vi "EyeTrackerFPGA (host).vi"() -> ()   [LabVIEW 2014]
uses:
  <vilib>/userdefined/High Color/nirio_resource_hc.ctl
  <instrlib>/niHWS/nihws.llb/niHWS Open File Permissions ID.ctl
  <vilib>/FPGAPlugInAG/PXI-7952R/niLvFpga_Open_PXI-7952R.vi
  <vilib>/rvi/interface/common/dynamic/niFpgaDynamicAddResources.vi
  <vilib>/FPGAPlugInAG/PXI-7954R/niLvFpga_Open_PXI-7954R.vi
  <vilib>/FPGAPlugInAG/PXI-7953R/niLvFpga_Open_PXI-7953R.vi
  <vilib>/FPGAPlugInAG/Dynamic/niLvFpga_Reset_Dynamic.vi
  <vilib>/Utility/error.llb/Error Cluster From Error Code.vi
  <vilib>/rvi/errors/niLvFpgaAdjustHostInterfaceError.vi
  <vilib>/FPGAPlugInAG/Dynamic/niLvFpga_Run_Dynamic.vi
  <vilib>/LabVIEW Targets/FPGA/FlexRIO/CustomFPGAMethods/79XXR_Method_IOModuleStatusImpl.vi
  <vilib>/rvi/interface/common/niFpgaWaitOnOcc.vi
  <vilib>/DAQmx/write.llb/DAQmx Write (Analog 1D DBL NChan 1Samp).vi
  <instrlib>/niHWS/nihws.llb/niHWS Write Digital U16.vi
  <vilib>/FPGAPlugInAG/Dynamic/niLvFpga_Close_Dynamic.vi
  <vilib>/rvi/interface/nirviOpenFPGA/nirviOpenFPGA.xnode
  FPGA Bitfiles/EyeTrackerFPGA_PXI-7952R_EyeTrackerFPGA(F_6273CC10.lvbitx
  FPGA Bitfiles/EyeTrackerFPGA_PXI-7954R_EyeTrackerFPGA-7_4D2D153E.lvbitx
  FPGA Bitfiles/EyeTrackerFPGA_FPGATarget_EyeTrackerFPGA-7_1NUruOWZ7TY_7953R.lvbitx
  <vilib>/rvi/interface/nirviMethod/nirviMethod.xnode
  <vilib>/rvi/interface/nirviReadWriteControl/nirviReadWriteControl.xnode
  <vilib>/rvi/interface/nirviCloseFPGA/nirviCloseFPGA.xnode
  <vilib>/rvi/errors/niLvFpgaMergeErrorWithErrorCode.vi
  <vilib>/rvi/interface/Simulation/niFpgaSimulationCallBeginRW.vi
  NiFpgaLv.dll
  <vilib>/FPGAPlugInAG/Dynamic/niLvFpga_ReadFifo_Dynamic.vi
  <vilib>/FPGAPlugInAG/Dynamic/niLvFpga_ConfigureFifo_Dynamic.vi
  <vilib>/FPGAPlugInAG/Dynamic/niLvFpga_StartFifo_Dynamic.vi
  <resource>/objmgr/daqmx.rc
panel:
  in  "Setup":u16(ring) items=["1", "2", "3"]
  out "Analog Output Error":errorcluster
  out "Select Setup":bool=TRUE
  in  "DA Output Task":refnum<k21>="OpticalTrackerOutWithPupilSize"
  in  "Raw  Image":bool=TRUE
  out "Frame Time (x10 ns)":u32
  out "TraceDisplayLoop":i32
  out "Frame Number":u32
  out "ImageDisplayLoop":i32
  out "Text File Write Error":errorcluster
  out "AVI Write Error":errorcluster
  in  "Image Acq Rate":dbl=20.0
  in  "Calibration":bool=TRUE
  in  "RIO Device":T1="RIO0"
  in  "MinUpdatePeriod":dbl=5.0
  out "Elements Remaining":u32
  in  "Record":bool
  out "Tracking":bool
  in  "Preview Thresh":dbl
  in  "AnalogOut":bool=TRUE
  out "UpdateRate":dbl
  out "TenFrameTime":u32
  in  "MonitorDelay":u32=100
  in  "FrameRate":dbl=250.0
  in  "Track":bool
  in  "Send":bool
  in  "Command":string
  in  "Viewing Rate":dbl=5.0
  in  "EyePosition.Shift":i8
  in  "Brighten":i32=1
  in  "Threshold":u32=2800
  out "RealRate":dbl
  out "DataAvailable":u32
  out "PushedToHost":u32
  out "PushedToMem":u32
  out "BufferToHost\\Full":bool
  out "Timed Out?":bool
  out "Acq Status.FrameWidth":u32
  out "Acq Status.FrameHeight":u32
  out "ImLoop":i32
  out "MonLoop":i32
  out "Acq Control.Grab":bool
  out "Grabbing":bool
  out "Grabbed":bool
  out "Acq Control.Acq":bool
  in  "Grab":bool=TRUE
  out "Waveform Chart":cluster{dbl, dbl, dbl}[](graph)
  out "Frame Width":u32
  in  "stopped":bool
  out "DMA Write Timeout?":bool
  out "I/O Enabled?":bool
  out "Frame Num":u32
  out "Frame Height":u32
  out "Image":T2(plugin-control)
  in  "stop":bool
  out "Initialized?":bool
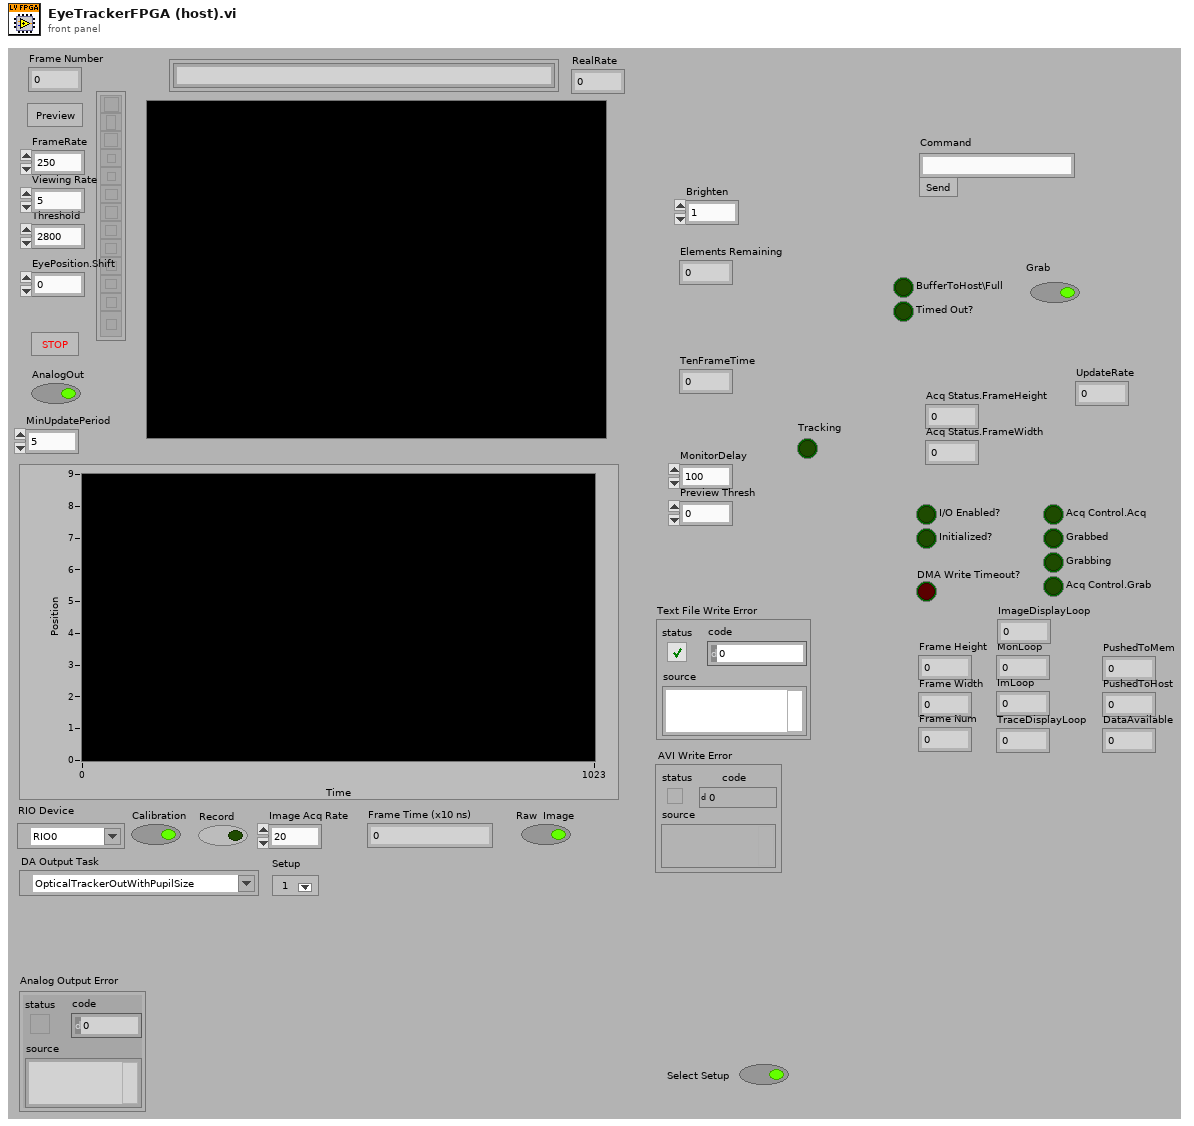
[diagram p1: front panel]
types:
  T1 = typedef "nirio_resource_hc.ctl" = tag
  T2 = typedef "IMAQ Image.ctl" = refnum<image>
  T3 = typedef "Image Type" = u32
  T4 = enum8{"Enabled", "Disabled", "Disabled and Grayed Out"}
  T5 = enum16{"open", "replace", "create", "open or create", "replace or create", "replace or create with confirmation"}
  T6 = typedef "niHWS Open File Permissions ID.ctl" = enum32{"Read Only", "Read/Write Existing", "Read/Write/Create New", "Read/Write/Create New Always"}
  T7 = typedef "AviRefnum.ctl" = refnum<k1>
  T8 = cluster{"Global Rectangle":i32[], "Contours":cluster{"Contour Type":u32, "ROI Type":u32, "Points":i32[]}[]}
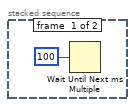
[diagram p2: hidden frame]
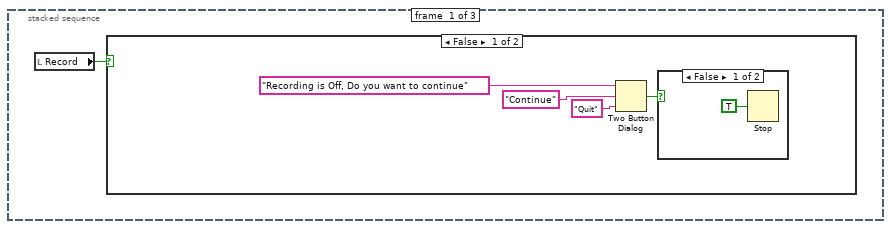
[diagram p3: hidden frame]
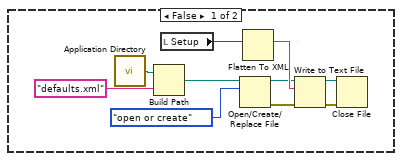
[diagram p6: hidden frame]
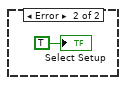
[diagram p7: hidden frame]
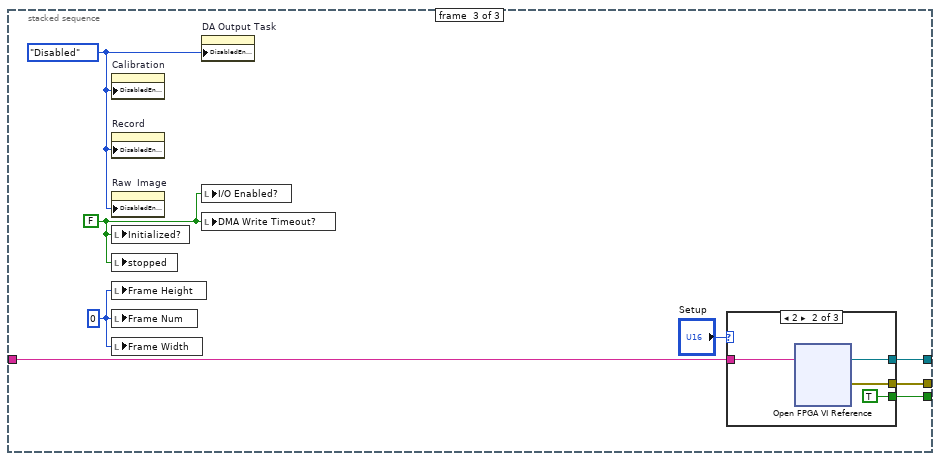
[diagram p9: hidden frame]
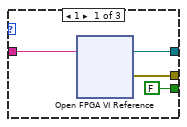
[diagram p10: hidden frame]
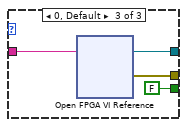
[diagram p11: hidden frame]
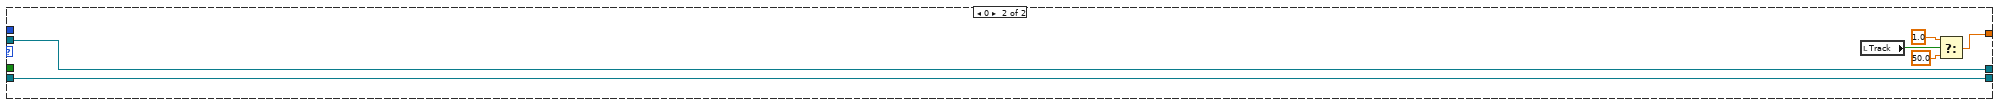
[diagram p20: hidden frame]
diagram:
  w13 = T3 0 items=["Grayscale (U8)", "Grayscale (I16)", "Grayscale (SGL)", "Complex (CSG)", "RGB (U32)", "HSL (U32)", "RGB (U64)", "Grayscale (U16)"] ("Image Type")
  w1 = T4."Enabled" ("Disabled")
  w88 = T3 0 items=["Grayscale (U8)", "Grayscale (I16)", "Grayscale (SGL)", "Complex (CSG)", "RGB (U32)", "HSL (U32)", "RGB (U64)", "Grayscale (U16)"] ("Image Type")
  # "To compile for S1:\nSelect the FPGA file from PXI-7954R\nSelect 10"
  # "relevant commands:\nsot 80 - 80 MB/s\nssf 500 - set frame rate\nset 5000 - set exposure time\nwse 0 1 x1 y1 x2 y2 - set window"
  # "Merge any errors.\nCleanup the image.\nClose the FPGA reference.\nDisplay any errors."
  # "Send software triggers as requested and monitor the acquisition status."
  # "Configure the trigger pulse width."
  # "Start the Serial Server for configuring the camera."
  # "Create the display image and set the bit depth to be 10 bits."
  # "Initialize the acquisition.  This will wait until a pixel clock is detected from the camera.  If the Initialized? indicater never lights up, make sure that the camera is connected properly."
  # "Wait for the Camera Link adapter module to be detected."
  # "Initialize the Host DMA FIFO."
  # "Configure the polarity of the Camera Link \nsignals.  This needs to be done prior to \nrunning the FPGA block diagram."
  # "Open a reference to the FPGA bitstream.\nInitialize the UI.\nReset the Flex RIO board."
  n1 = local write "Track"(FALSE ("Track")) -> ()
  n2 = local write "Tracking"(FALSE ("Tracking")) -> ()
  n3 = stacked-sequence {
    tunnel: [_ _ w136] -> w78
    tunnel: [_ _ w130] -> w47
    tunnel: [_ _ w133] -> w30
    tunnel: "RIO Device" -> [_ _ w132]
    frame #0 {
      n4 = local read "Record"() -> (w93:bool)
      n5 = case shown="False" w93 {
        frame False {
          n6 = Two Button Dialog(message="Recording is Off, Do you want to continue", 1:"Quit" ("F button name (\"Cancel\")"), 2:"Continue" ("T button name (\"OK\")")) -> (T button?=w94:bool)
          n7 = case shown="False" w94 {
            frame False {
              n8 = Stop(stop? (T)=TRUE) -> ()
            }
            frame True {
            }
          }
        }
        frame True {
        }
      }
    }
    frame #1 {
      n9 = call <vilib>:"Application Directory.vi"() -> ("Application Directory"=w102:path)
      n10 = Build Path(base path=w102, name or relative path="defaults.xml") -> (appended path=w100:path)
      n11 = call <vilib>:"Check if File or Folder Exists.vi"("path"=w100) -> ("error out"=w99:errorcluster, "file or folder exists?"=w101:bool)  [unwired: 8 in, 1 out]
      n12 = case shown="True" w101 {
        tunnel: w100 -> [_ w115]
        tunnel: w99 -> [_ w114]
        frame False {
          n13 = call <vilib>:"Application Directory.vi"() -> ("Application Directory"=w112:path)
          n14 = Build Path(base path=w112, name or relative path="defaults.xml") -> (appended path=w113:path)
          n15 = local read "Setup"() -> (w104:u16)
          n16 = Open/Create/Replace File(file path (use dialog)=w113, operation (0:open)=T5."open or create") -> (refnum out=w106:refnum<file>, error out=w108:errorcluster)  [unwired: 4 in, 1 out]
          n17 = Flatten To XML(anything=w104) -> (xml string=w107:string)
          n18 = Write to Text File(file (use dialog)=w106, text=w107, error in=w108) -> (refnum out=w110:refnum<file>, error out=w111:errorcluster)  [unwired: 1 in, 1 out]
          n19 = Close File(refnum=w110, error in=w111) -> ()  [unwired: 2 out]
        }
        frame True {
          n20 = case shown="No Error" w114 {
            selector: w114 -> [w121 _]
            tunnel: w115 -> [w124 _]
            frame No Error {
              n21 = Read from Text File(file (use dialog)=w124, error in=w121) -> (refnum out=w122:refnum<file>, text=w120:string, error out=w123:errorcluster)  [unwired: 2 in, 1 out]
              n22 = Close File(refnum=w122, error in=w123) -> (error out=w119:errorcluster)  [unwired: 1 out]
              n23 = Unflatten From XML(xml string=w120, type=u16 0, error in (no error)=w119) -> (value=w116:u16, error out=w117:errorcluster)
              n24 = case shown="No Error" w117 {
                selector: w117 -> [w127 _]
                tunnel: w116 -> [w126 _]
                frame No Error {
                  n25 = Variant To Data(error in=w127, Variant=w126) -> (data=w125:u16)  [unwired: 1 in, 1 out]
                  n26 = local write "Setup"(w125) -> ()
                }
                frame Error {
                  "Select Setup" <- TRUE ("Select Setup")
                }
              }
            }
            frame Error {
            }
          }
        }
      }
    }
    frame #2 {
      w131 = T4."Disabled" ("Disabled")
      w135 = u32 0 ("Num Lines Acq'd")
      w134 = FALSE ("stop")
      n27 = property on="Calibration" class="Bool (strict)"("DisabledEnum"=w131) -> ()  [unwired: 2 in, 2 out]
      n28 = property on="Record" class="Bool (strict)"("DisabledEnum"=w131) -> ()  [unwired: 2 in, 2 out]
      n29 = property on="Raw  Image" class="Bool (strict)"("DisabledEnum"=w131) -> ()  [unwired: 2 in, 2 out]
      n30 = local write "Initialized?"(w134) -> ()
      n31 = local write "stopped"(w134) -> ()
      n32 = local write "Frame Height"(w135) -> ()
      n33 = local write "Frame Num"(w135) -> ()
      n34 = local write "Frame Width"(w135) -> ()
      n35 = property on="DA Output Task" class="DAQmxName (strict)"("DisabledEnum"=w131) -> ()  [unwired: 2 in, 2 out]
      n36 = local write "I/O Enabled?"(w134) -> ()
      n37 = local write "DMA Write Timeout?"(w134) -> ()
      n38 = case shown="2" "Setup" {
        tunnel: [w140 w143 w148] -> w136
        tunnel: [w139 w142 w146] -> w130
        tunnel: w132 -> [w138 w144 w145]
        tunnel: [FALSE TRUE FALSE] -> w133
        frame 1 {
          n39 = xnode "Open FPGA VI Reference"("resource name"=w138) -> ("FPGA VI Reference Out"=w140:refnum<k20>, "error out"=w139:errorcluster)  [unwired: 1 in]
        }
        frame 2 {
          n40 = xnode "Open FPGA VI Reference"("resource name"=w144) -> ("FPGA VI Reference Out"=w143:refnum<k20>, "error out"=w142:errorcluster)  [unwired: 1 in]
        }
        frame 0, Default {
          n41 = xnode "Open FPGA VI Reference"("resource name"=w145) -> ("FPGA VI Reference Out"=w148:refnum<k20>, "error out"=w146:errorcluster)  [unwired: 1 in]
        }
      }
    }
  }
  n42 = xnode "Invoke Method"("FPGA VI Reference In"=w78, "error in"=w47) -> ("FPGA VI Reference Out"=w32:refnum<k20>, "error out"=w66:errorcluster)
  n43 = xnode "Read/Write Control"("FPGA VI Reference In"=w32, "error in"=w66, "IO Module Config.CL FVAL Active High"=TRUE, "IO Module Config.CL LVAL Active High"=TRUE, "IO Module Config.CL DVAL Active High"=TRUE, "IO Module Config.CL Spare Active High"=TRUE, "Acq Control.Grab"=FALSE, "10-bit"=w30, "EyePosition.Color"="Raw  Image") -> ("FPGA VI Reference Out"=w67:refnum<k20>, "error out"=w65:errorcluster)
  n44 = xnode "Invoke Method"("FPGA VI Reference In"=w67, "error in"=w65) -> ("FPGA VI Reference Out"=w79:refnum<k20>, "error out"=w31:errorcluster)  [unwired: 1 in]
  n45 = call <vilib>:"Simple Error Handler.vi"("error in (no error)"=w31) -> ()  [unwired: 4 in, 5 out]
  n46 = while {
    tunnel: w79 -> [w149]
    tunnel: [w152] -> w51
    tunnel: w31 -> [w153]
    tunnel: [w151] -> w59
    i -> [w155]
    stop <- w160 stop-if-true
    # "An error is returned and VI execution is stopped if the IO Module has not become initialized after 1 second."
    n47 = xnode "Invoke Method"("FPGA VI Reference In"=w149, "error in"=w153) -> ("FPGA VI Reference Out"=w152:refnum<k20>, "error out"=w151:errorcluster, "IO Enabled?"=w150:bool)  [unwired: 3 out]
    n48 = Wait (ms)(milliseconds to wait=u32 10) -> ()  [unwired: 1 out]
    n49 = Greater Or Equal?(x=w155, y=100) -> (x >= y?=w157:bool)
    n50 = case shown="True" w157 {
      tunnel: [w163 FALSE ("Configured?")] -> w154
      tunnel: w150 -> [w163 _]
      tunnel: w151 -> [w162 w164]
      tunnel: [w162 w166] -> w156
      frame False {
      }
      frame True {
        n51 = Merge Errors(w164, errorcluster {"status"=TRUE, "code"=-8999, "source"="IO Module not initialized before the specified timeout."} ("error in")) -> (w166:errorcluster)
      }
    }
    "I/O Enabled?" <- w154
    n52 = Unbundle By Name(w156) -> ("status"=w161:bool)
    n53 = Or(x=w161, y=w154) -> (x .or. y?=w160:bool)
  }
  n54 = xnode "Invoke Method"("FPGA VI Reference In"=w51, "error in"=w59, "Requested Depth"=u32 10000 ("Depth")) -> ("FPGA VI Reference Out"=w57:refnum<k20>, "error out"=w56:errorcluster)  [unwired: 1 out]
  n55 = Multiply(x=u32 1400 ("Image Height"), y=u32 1024 ("Image Height")) -> (x*y=w39:u32)
  n56 = xnode "Invoke Method"("FPGA VI Reference In"=w57, "error in"=w56) -> ("FPGA VI Reference Out"=w55:refnum<k20>, "error out"=w54:errorcluster)
  n57 = Divide(x=w39, y=u32 2 ("Image Height")) -> (x/y=w37:dbl)
  n58 = xnode "Invoke Method"("FPGA VI Reference In"=w55, "error in"=w54, "Requested Depth"=w37) -> ("FPGA VI Reference Out"=w77:refnum<k20>, "error out"=w76:errorcluster)  [unwired: 1 out]
  n59 = xnode "Invoke Method"("FPGA VI Reference In"=w77, "error in"=w76) -> ("FPGA VI Reference Out"=w75:refnum<k20>, "error out"=w74:errorcluster)
  n60 = xnode "Read/Write Control"("FPGA VI Reference In"=w75, "error in"=w74, "Acq Control.Initialize"=TRUE ("Arm Acquisition")) -> ("FPGA VI Reference Out"=w91:refnum<k20>, "error out"=w90:errorcluster)
  n61 = while {
    tunnel: w91 -> [w180]
    tunnel: w90 -> [w179]
    tunnel: [w178] -> w6
    tunnel: [w170] -> _
    i -> [w173]
    stop <- w177 stop-if-true
    # "An error is returned and VI execution is stopped if the acquisition has not become initialized after 1 second."
    n62 = xnode "Read/Write Control"("FPGA VI Reference In"=w180, "error in"=w179) -> ("FPGA VI Reference Out"=w178:refnum<k20>, "error out"=w171:errorcluster, "Acq Status.Initialized"=w169:bool)
    n63 = Wait (ms)(milliseconds to wait=u32 10) -> ()  [unwired: 1 out]
    n64 = Greater Or Equal?(x=w173, y=100) -> (x >= y?=w172:bool)
    n65 = case shown="False" w172 {
      tunnel: [w182 FALSE ("Configured?")] -> w168
      tunnel: w169 -> [w182 _]
      tunnel: w171 -> [w181 w183]
      tunnel: [w181 w185] -> w170
      frame False {
      }
      frame True {
        n66 = Merge Errors(w183, errorcluster {"status"=TRUE, "code"=-8999, "source"="Acquisition not initialized before the specified timeout."} ("error in")) -> (w185:errorcluster)
      }
    }
    "Initialized?" <- w168
    n67 = Unbundle By Name(w170) -> ("status"=w176:bool)
    n68 = Or(x=w176, y=w168) -> (x .or. y?=w177:bool)
  }
  n69 = case shown="True" "Record" {
    tunnel: [_ w195] -> w44
    tunnel: [_ w203] -> w42
    tunnel: [_ w202] -> w15
    tunnel: [_ w190] -> w17
    frame False {
    }
    frame True {
      n70 = call "File Dialog"() -> ("selected path"=w201:path)  [unwired: 12 in, 3 out]
      n71 = Strip Path(path=w201) -> (stripped path=w192:path, name=w194:string)
      n72 = Concatenate Strings(w194, ".h5" ("name or relative path")) -> (w199:string)
      n73 = Concatenate Strings(w194, ".txt" ("string")) -> (w193:string)
      n74 = Concatenate Strings(w194, ".avi" ("string")) -> (w197:string)
      n75 = Build Path(base path=w192, name or relative path=w199) -> (appended path=w210:path)
      n76 = Build Path(base path=w192, name or relative path=w193) -> (appended path=w191:path)
      n77 = Build Path(base path=w192, name or relative path=w197) -> (appended path=w196:path)
      n78 = call <instrlib>:"niHWS Open File.vi"("permissions (0:read only)"=niHWS_Open_File_Permissions_ID."Read/Write/Create New Always", "file path"=w210) -> ("error out"=w207:errorcluster, "file handle"=w208:u32)  [unwired: 8 in]
      n79 = call <instrlib>:"niHWS New Wfm Reference.vi"("compression level (0:none)"=0, "error in (no error)"=w207, "waveform name (empty)"="EyeTraces", "group name (empty)"="EyeTraces", "file handle in"=w208) -> ("waveform reference"=w203:u32, "file handle out"=w202:u32)  [unwired: 4 in, 1 out]
      n80 = Open/Create/Replace File(file path (use dialog)=w191, operation (0:open)=T5."create", access (0:read/write)=enum16{"read/write", "read-only", "write-only"}."read/write") -> (refnum out=w190:refnum<file>)  [unwired: 3 in, 2 out]
      n81 = call "OpenAVIFile.vi"("AVI Path"=w196) -> ("Avi Refnum"=w195:T7)  [unwired: 9 in, 1 out]
    }
  }
  n82 = call <vilib>:"DAQmx Create Task.vi"("task to copy"="DA Output Task") -> ("task out"=w29:refnum<k21>, "error out"=w28:errorcluster)  [unwired: 13 in]
  n83 = case shown="False" "Calibration" {
    tunnel: w29 -> [w214 w215]
    tunnel: w28 -> [w213 _]
    tunnel: [w212 w215] -> w27
    frame False {
      n84 = property class="DAQmx Timing"(reference=w214, error in=w213, "RefClk.Src"=tag "/Dev3/PXI_Clk10") -> (reference out=w212:refnum<k21>)  [unwired: 1 out]
    }
    frame True {
    }
  }
  n85 = call "WriteStringUART.vi"("String"="\rsot 80\rsot 80\rwse 0 1 0 0 1400 1024\r\nset 20000\r\nssf 50\r\n", "FPGA VI Reference In"=w6) -> ("error out"=w8:errorcluster, "FPGA VI Reference Out"=w49:refnum<k20>)  [unwired: 8 in]
  n86 = Multiply(x=u32 40, y=u32 100 ("Trigger Pulse Width (us)")) -> (x*y=w71:u32)
  n87 = xnode "Read/Write Control"("FPGA VI Reference In"=w49, "Trigger.Trigger Pulse Width (40 MHz Ticks)"=w71, "Acq Control.Acq"=TRUE, "EyePosition.Send"=FALSE, "EyePosition.Threshold"=u16 0) -> ("FPGA VI Reference Out"=w48:refnum<k20>, "error out"=w86:errorcluster)  [unwired: 1 in]
  n88 = call "IMAQ Create"("Image Name"="I16 Image", "Image Type"=w88, "error in (no error)"=w8) -> ("New Image"=w21:T2, "error out"=w7:errorcluster)  [unwired: 2 in]
  n89 = Obtain Queue(element data type=cluster{dbl, dbl, dbl} {0.0, 0.0, 0.0} ("output cluster"), error in (no error)=w7) -> (queue out=w34:refnum<queue>)  [unwired: 3 in, 2 out]
  n90 = Obtain Queue(max queue size (-1, unlimited)=1, name (unnamed)="Image Display Queue", element data type=w21) -> (queue out=w19:refnum<queue>)  [unwired: 2 in, 2 out]
  n91 = call "IMAQ Create"("Image Name"="SavedImage", "Image Type"=w13) -> ("New Image"=w10:T2)  [unwired: 3 in, 1 out]
  n92 = Merge Errors(w86, w7) -> (w85:errorcluster)
  n93 = while {
    tunnel: w34 -> [w219]
    i -> [w216]
    stop <- w220 stop-if-true
    n94 = Flush Queue(queue=w219) -> (remaining elements=→"Waveform Chart":cluster{dbl, dbl, dbl}[])  [unwired: 1 in, 2 out]
    n95 = Wait Until Next ms Multiple(millisecond multiple=u32 100) -> ()  [unwired: 1 out]
    n96 = local read "stopped"() -> (w220:bool)
    "TraceDisplayLoop" <- w216
  }
  n97 = while "Display Image Frames at Viewing Rate" {
    tunnel: w19 -> [w227]
    i -> [w222]
    stop <- w221 stop-if-true
    n98 = local read "stopped"() -> (w221:bool)
    n99 = case shown="False" w221 {
      tunnel: w227 -> [w231 _]
      frame False {
        n100 = Preview Queue Element(queue=w231, timeout in ms (-1)=1) -> (element=w229:T2, timed out?=w230:bool)  [unwired: 1 in, 2 out]
        n101 = case shown="False" w230 {
          tunnel: w229 -> [w232 _]
          frame False {
            "Image" <- w232
          }
          frame True {
          }
        }
      }
      frame True {
      }
    }
    n102 = Reciprocal(x="Viewing Rate") -> (1/x=w226:dbl)
    n103 = Multiply(x=w226, y=1000.0) -> (x*y=w223:dbl)
    n104 = Wait Until Next ms Multiple(millisecond multiple=w223) -> ()  [unwired: 1 out]
    "ImageDisplayLoop" <- w222
  }
  n105 = while {
    tunnel: w27 -> [w247]
    tunnel: [w246] -> w45
    tunnel: "Record" -> [w244]
    tunnel: w42 -> [w245]
    shift-right: [w239] -> _
    shift-left: w48 -> [w242]
    tunnel: w34 -> [w233]
    stop <- w248 stop-if-true
    n106 = xnode "Invoke Method"("FPGA VI Reference In"=w242, "Number of Elements"=0 ("IRQ Number(s)"), "Timeout (ms)"=0) -> ("FPGA VI Reference Out"=w240:refnum<k20>, "Elements Remaining"=w238:u32)  [unwired: 1 in, 2 out]
    n107 = case shown="1, Default" w238 {
      selector: w238 -> [w266 _]
      tunnel: w247 -> [w250 w338]
      tunnel: [w274 w338] -> w246
      tunnel: w244 -> [w273 _]
      tunnel: w245 -> [w272 _]
      tunnel: w240 -> [w271 w337]
      tunnel: [w268 w337] -> w239
      tunnel: [w260 w334] -> w236
      tunnel: w233 -> [w263 _]
      frame 1, Default {
        n108 = xnode "Invoke Method"("FPGA VI Reference In"=w271, "Number of Elements"=w266, "Timeout (ms)"=1) -> ("FPGA VI Reference Out"=w268:refnum<k20>, "Data"=w259:u64[], "Elements Remaining"=→"Elements Remaining":u32)  [unwired: 1 in, 1 out]
        n109 = Tick Count (ms)() -> (millisecond timer value=w277:u32)
        n110 = feedback-in #1(w277) -> ()
        n111 = feedback #1() -> (w280:u32)  [unwired: 1 in]
        n112 = case shown="True" w273 {
          tunnel: w259 -> [_ w325]
          tunnel: w272 -> [_ w326]
          frame False {
          }
          frame True {
            n113 = Split Number(x=w325) -> (hi(x)=w324:u32[], lo(x)=w321:u32[])
            n114 = Split Number(x=w324) -> (hi(x)=w323:u16[], lo(x)=w322:u16[])
            n115 = Split Number(x=w321) -> (hi(x)=w320:u16[], lo(x)=w319:u16[])
            n116 = Interleave 1D Arrays(w323, w322) -> (w318:u16[])
            n117 = Interleave 1D Arrays(w320, w319) -> (w317:u16[])
            n118 = Interleave 1D Arrays(w318, w317) -> (w316:u16[])
            n119 = call-poly <instrlib>:"niHWS Write.vi"("data"=w316, "waveform reference in"=w326) -> ()  [unwired: 8 in, 2 out]
          }
        }
        n120 = Subtract(x=w277, y=w280) -> (x-y=w279:u32)
        n121 = for {
          tunnel: w263 -> [w304]
          tunnel: w259 -> [w299] mode=indexing
          tunnel: [w300] -> w258
          border: dbl[] [0.0, 0.0] -> [_]
          shift-right: [w287] -> w252
          shift-left: 0.0 -> [w288]
          w285 = 32768
          w290 = -10
          w291 = 10
          w295 = 0.5
          w293 = 20
          n122 = Split Number(x=w299) -> (hi(x)=w298:u32, lo(x)=w297:u32)
          n123 = Split Number(x=w297) -> (hi(x)=w286:u16)  [unwired: 1 out]
          n124 = Split Number(x=w298) -> (hi(x)=w310:u16, lo(x)=w309:u16)
          n125 = Divide(x=w310, y=w285) -> (x/y=w315:dbl)
          n126 = Divide(x=w309, y=w285) -> (x/y=w314:dbl)
          n127 = Divide(x=w286, y=w285) -> (x/y=w296:dbl)
          n128 = Build Array(w315, w314) -> (w313:dbl[])
          n129 = Subtract(x=w296, y=w295) -> (x-y=w294:dbl)
          n130 = Subtract(x=w313, y=w295) -> (x-y=w312:dbl[])
          n131 = Multiply(x=w312, y=w293) -> (x*y=w311:dbl[])
          n132 = Multiply(x=w294, y=w293) -> (x*y=w292:dbl)
          n133 = In Range and Coerce(upper limit=w291, x=w311, lower limit=w290) -> (coerced(x)=w302:dbl[])  [unwired: 1 out]
          n134 = shared-variable "My Computer\\Shared Variables.lvlib\\EyePosition"(w302) -> ()  [unwired: 1 in, 1 out]
          n135 = In Range and Coerce(upper limit=w291, x=w292, lower limit=w290) -> (coerced(x)=w289:dbl)  [unwired: 1 out]
          n136 = feedback #2() -> (w301:dbl[])
          n137 = Add(x=w302, y=w301) -> (x+y=w300:dbl[])
          n138 = feedback-in #2(w300) -> ()
          n139 = Index Array(array=w302, index #1=0 ("index"), index #2=1 ("index")) -> (element #1=w306:dbl, element #2=w305:dbl)
          n140 = Add(x=w289, y=w288) -> (x+y=w287:dbl)
          n141 = Bundle(w306, w305, w289) -> (w303:cluster{dbl, dbl, dbl})  [unwired: 1 in]
          n142 = Enqueue Element(queue=w304, element=w303) -> ()  [unwired: 2 in, 3 out]
        }
        n143 = Divide(x=w279, y=u32 20000) -> (x/y=w267:dbl)
        n144 = Reciprocal(x=w267) -> (1/x=→"UpdateRate":dbl)
        n145 = property on="Hack to allow 2 channel and 3 channel tasks from the same program" class="DAQmx Task"(reference=w250) -> ("NumChans"=w249:u32)  [unwired: 1 in, 2 out]
        n146 = Array Size(array=w259) -> (size(s)=w256:i32)
        n147 = Divide(x=w252, y=w256) -> (x/y=w251:dbl)
        n148 = Divide(x=w258, y=w256) -> (x/y=w255:dbl[])
        n149 = case shown="3" w249 {
          tunnel: w255 -> [w281 w284]
          tunnel: [w281 w283] -> w254
          tunnel: w251 -> [_ w282]
          frame 2, Default {
          }
          frame 3 {
            n150 = Build Array (concatenate)(w284, w282) -> (w283:dbl[])
          }
        }
        n151 = local read "RealRate"() -> (w262:dbl)
        n152 = Reciprocal(x=w262) -> (1/x=w261:dbl)
        n153 = case shown="True" "AnalogOut" {
          tunnel: w250 -> [w327 w332]
          tunnel: [w327 w331] -> w274
          tunnel: w254 -> [_ w329]
          frame False {
          }
          frame True {
            n154 = call-poly <vilib>:"DAQmx Write.vi"("task/channels in"=w332, "auto start"=TRUE, "data"=w329) -> ("task out"=w331:refnum<k21>, "error out"=→"Analog Output Error":errorcluster)  [unwired: 10 in, 1 out]
          }
        }
        n155 = Multiply(x=1000.0, y=w261) -> (x*y=w264:dbl)
        n156 = Decrement(x=w264) -> (x-1=w260:dbl)
      }
      frame 0 {
        n157 = local read "Track"() -> (w336:bool)
        n158 = Select(t=1.0, s=w336, f=50.0) -> (s? t:f=w334:dbl)
      }
    }
    n159 = In Range and Coerce(upper limit=200.0, x=w236, lower limit="MinUpdatePeriod") -> (coerced(x)=w237:dbl)  [unwired: 1 out]
    n160 = local read "stopped"() -> (w248:bool)
    n161 = Wait Until Next ms Multiple(millisecond multiple=w237) -> ()  [unwired: 1 out]
  }
  n162 = while {
    tunnel: w48 -> [w351]
    tunnel: w85 -> [_]
    tunnel: w21 -> [w361]
    tunnel: [w350] -> w69
    tunnel: [w359] -> w87
    tunnel: [w354] -> w82
    tunnel: w44 -> [w347]
    tunnel: "Record" -> [w346]
    shift-right: [w353] -> w18
    shift-left: w19 -> [w355]
    tunnel: w17 -> [w349]
    tunnel: [w344] -> w16
    tunnel: w10 -> [w348]
    tunnel: [w345] -> w12
    tunnel: [w343] -> w11
    tunnel: [w342] -> w9
    i -> [w362]
    stop <- w360 stop-if-true
    # "Acquire a single frame as requested.\nUse the width and height to determine how much data to read from the DMA FIFO.\nConvert the data into a Vision Image for display.\nAdd post processiong steps as needed."
    n163 = local read "Track"() -> (w341:bool)
    n164 = feedback-in #3(w341) -> ()
    n165 = feedback #3() -> (w340:bool)  [unwired: 1 in]
    n166 = Equal?(x=w341, y=w340) -> (x = y?=w339:bool)
    n167 = Compound Arithmetic op=AND(w346, w341, w339) -> (w345:bool)
    n168 = stacked-sequence "Transfer Image Frame From fPGA to Host" {
      seq-local: [_ w380 _] -> [_ _ w483]
      tunnel: w351 -> [w365 w387 w484]
      tunnel: w361 -> [_ w382 _]
      tunnel: [_ w381 _] -> w354
      tunnel: [_ _ w485] -> w360
      tunnel: [_ _ w482] -> w350
      tunnel: [_ _ w480] -> w359
      tunnel: w349 -> [_ w377 _]
      tunnel: w348 -> [_ w376 _]
      tunnel: w347 -> [_ w375 _]
      tunnel: w345 -> [_ w374 _]
      tunnel: [_ w373 _] -> w344
      tunnel: [_ w372 _] -> w343
      tunnel: [_ w371 _] -> w342
      frame #0 {
        n169 = xnode "Read/Write Control"("FPGA VI Reference In"=w365, "Acq Control.Grab"="Grab") -> ("FPGA VI Reference Out"=w364:refnum<k20>)  [unwired: 1 in, 1 out]
        n170 = for {
          N: 100 -> [_]
          tunnel: w364 -> [w370]
          tunnel: [w369] -> _
          stop <- w368 continue-if-true
          n171 = xnode "Read/Write Control"("FPGA VI Reference In"=w370) -> ("FPGA VI Reference Out"=w369:refnum<k20>, "Grabbing"=w368:bool)  [unwired: 1 in, 1 out]
          n172 = Wait Until Next ms Multiple(millisecond multiple=u32 1) -> ()  [unwired: 1 out]
        }
      }
      frame #1 {
        n173 = xnode "Read/Write Control"("FPGA VI Reference In"=w387) -> ("FPGA VI Reference Out"=w386:refnum<k20>, "error out"=w385:errorcluster, "Acq Status.FrameHeight"=w378:u32, "Acq Status.FrameWidth"=w384:u32, "Grabbed"=w383:bool)  [unwired: 1 in]
        n174 = case shown="True" w383 {
          tunnel: w382 -> [w392 w453]
          tunnel: [w391 w452] -> _
          tunnel: [_ w451] -> w380
          tunnel: [w392 w450] -> w381
          tunnel: w386 -> [w391 w449]
          tunnel: w385 -> [_ w448]
          tunnel: w378 -> [_ w444]
          tunnel: w384 -> [_ w443]
          tunnel: "Brighten" -> [_ w433]
          tunnel: w374 -> [_ w415]
          tunnel: w377 -> [w390 w421]
          tunnel: w376 -> [w388 w419]
          tunnel: w375 -> [w389 w418]
          tunnel: [w390 w417] -> w373
          tunnel: [w389 w416] -> w372
          tunnel: [w388 w413] -> w371
          frame False {
          }
          frame True {
            w403 = 0 ("index (row)")
            n175 = Multiply(x=w444, y=w443) -> (x*y=w437:u32)
            n176 = Divide(x=w437, y=2.0) -> (x/y=w435:dbl)
            n177 = xnode "Invoke Method"("FPGA VI Reference In"=w449, "error in"=w448, "Number of Elements"=w435, "Timeout (ms)"=500) -> ("FPGA VI Reference Out"=w442:refnum<k20>, "error out"=w441:errorcluster, "Data"=w434:u16[], "Elements Remaining"=w439:u32)
            n178 = xnode "Invoke Method"("FPGA VI Reference In"=w442, "error in"=w441, "Number of Elements"=w439) -> ("FPGA VI Reference Out"=w452:refnum<k20>, "error out"=w440:errorcluster)  [unwired: 1 in, 2 out]
            n179 = Split Number(x=w434) -> (hi(x)=w447:u8[], lo(x)=w446:u8[])
            n180 = local read "Setup"() -> (w393:u16)
            n181 = Interleave 1D Arrays(w447, w446) -> (w445:u8[])
            n182 = Reshape Array(w445, w444, w443) -> (w428:u8[][])
            n183 = case shown="2" w393 {
              tunnel: [640.0 ("x") 1400.0 ("x")] -> w410
              tunnel: [480.0 ("y") 1024.0 ("y")] -> w409
              frame 0, 1, Default {
              }
              frame 2 {
              }
            }
            n184 = Multiply(x=w433, y=w428) -> (x*y=w412:i32[][])
            n185 = Array Size(array=w412) -> (size(s)=w411:i32[])
            n186 = Index Array(array=w428, index (row) #1=w403, index (col) #1=4 ("disabled index (col)"), index (row) #2=w403, index (col) #2=5 ("disabled index (col)"), index (row) #3=w403, index (col) #3=2 ("disabled index (col)"), index (row) #4=w403, index (col) #4=3 ("disabled index (col)"), index (row) #5=w403, index (col) #5=8 ("disabled index (col)"), index (row) #6=w403, index (col) #6=9 ("disabled index (col)"), index (row) #7=w403, index (col) #7=6 ("disabled index (col)"), index (row) #8=w403, index (col) #8=7 ("disabled index (col)")) -> (element #1=w429:u8, element #2=w430:u8, element #3=w425:u8, element #4=w424:u8, element #5=w400:u8, element #6=w399:u8, element #7=w398:u8, element #8=w397:u8)
            n187 = Join Numbers(hi=w429, lo=w430) -> ((hi.lo)=w423:u16)
            n188 = Join Numbers(hi=w425, lo=w424) -> ((hi.lo)=w422:u16)
            n189 = Join Numbers(hi=w400, lo=w399) -> ((hi.lo)=w396:u16)
            n190 = Join Numbers(hi=w398, lo=w397) -> ((hi.lo)=w395:u16)
            n191 = Multiply Array Elements(1:w411) -> (0:w407:i32)
            n192 = Multiply(x=w410, y=w409) -> (x*y=w408:dbl)
            n193 = Join Numbers(hi=w423, lo=w422) -> ((hi.lo)=w420:u32)
            "Frame Number" <- w420
            n194 = Join Numbers(hi=w396, lo=w395) -> ((hi.lo)=w394:u32)
            "Frame Time (x10 ns)" <- w394
            n195 = Not Equal?(x=w407, y=w408) -> (x != y?=w406:bool)
            n196 = And(x=w415, y=w406) -> (x .and. y?=w414:bool)
            n197 = case "Store in File" shown="True" w414 {
              tunnel: w418 -> [w460 w479]
              tunnel: [w460 w471] -> w416
              tunnel: w421 -> [w459 w478]
              tunnel: w420 -> [_ w473]
              tunnel: [w459 w477] -> w417
              tunnel: w419 -> [w458 w472]
              tunnel: w412 -> [_ w469]
              tunnel: [w458 w466] -> w413
              tunnel: w394 -> [_ w465]
              frame False {
              }
              frame True {
                n198 = To Unsigned Byte Integer(number=w469) -> (unsigned 8bit integer=w470:u8[][])
                n199 = Number To Decimal String(number=w473) -> (decimal integer string=w476:string)  [unwired: 1 in]
                n200 = Number To Decimal String(number=w465) -> (decimal integer string=w464:string)  [unwired: 1 in]
                n201 = call "IMAQ ArrayToImage"("Image Pixels (U8)"=w470, "Image"=w472) -> ("error out"=w468:errorcluster, "Image Out"=w466:T2)  [unwired: 8 in]
                n202 = call "IMAQ AVI Write Frame"("error in (no error)"=w468, "Image"=w466, "Avi Refnum"=w479) -> ("error out"=→"AVI Write Error":errorcluster, "Avi Refnum (duplicate)"=w471:T7)  [unwired: 7 in]
                n203 = Concatenate Strings(w476, "\t", w464, "\r", "\n") -> (w475:string)
                n204 = Write to Text File(file (use dialog)=w478, text=w475) -> (refnum out=w477:refnum<file>, error out=→"Text File Write Error":errorcluster)  [unwired: 2 in, 1 out]
              }
            }
            n205 = call "IMAQ ArrayToImage"("error in (no error)"=w440, "Image Pixels (U8)"=w412, "Image"=w453) -> ("error out"=w451:errorcluster, "Image Out"=w450:T2)  [unwired: 7 in]
          }
        }
      }
      frame #2 {
        n206 = local read "stopped"() -> (w486:bool)
        n207 = xnode "Read/Write Control"("FPGA VI Reference In"=w484, "error in"=w483, "Grabbed"=FALSE) -> ("FPGA VI Reference Out"=w480:refnum<k20>, "error out"=w482:errorcluster)
        n208 = Compound Arithmetic op=OR("stop", w486) -> (w485:bool)
        n209 = local write "stopped"(w485) -> ()
        n210 = Unbundle By Name(w482) -> ()  [unwired: 1 out]
        n211 = xnode "Read/Write Control"("FPGA VI Reference In"=w480, "Grabbed"=FALSE) -> ()  [unwired: 1 in, 2 out]
      }
    }
    n212 = Reciprocal(x="Image Acq Rate") -> (1/x=w358:dbl)
    n213 = Multiply(x=w358, y=1000.0) -> (x*y=w356:dbl)
    n214 = Wait Until Next ms Multiple(millisecond multiple=w356) -> ()  [unwired: 1 out]
    n215 = Lossy Enqueue Element(queue=w355, element=w354) -> (queue out=w353:refnum<queue>)  [unwired: 1 in, 3 out]
    "ImLoop" <- w362
  }
  n216 = while {
    tunnel: w48 -> [w526]
    tunnel: [w521] -> w68
    i -> [w514]
    stop <- w520 stop-if-true
    n217 = Boolean To (0,1)(Boolean=TRUE) -> (0, 1=w501:i16)
    n218 = local read "RealRate"() -> (w499:dbl)
    n219 = Multiply(x=w501, y="Threshold") -> (x*y=w500:u32)
    n220 = Wait Until Next ms Multiple(millisecond multiple="MonitorDelay") -> ()  [unwired: 1 out]
    n221 = Divide(x=w500, y=w499) -> (x/y=w493:dbl)
    n222 = local read "Tracking"() -> (w490:bool)
    n223 = Select(t=w493, s=w490, f="Preview Thresh") -> (s? t:f=w494:dbl)
    n224 = xnode "Read/Write Control"("FPGA VI Reference In"=w526, "Trigger.Send Software Trigger"=FALSE ("Software Trigger"), "EyePosition.Threshold"=w494, "EyePosition.Shift"="EyePosition.Shift", "EyePosition.Send"="Track") -> ("error out"=w522:errorcluster, "Acq Status.Acq'd Frame Height"=→"Frame Height":u32, "Acq Status.Frames Acq'd"=→"Frame Num":u32, "Acq Status.Acq'd Frame Width"=→"Frame Width":u32, "Acq Status.DMA Write Timeout"=w511:bool, "Acq Control.Acq"=→"Acq Control.Acq":bool, "Grabbed"=→"Grabbed":bool, "Grabbing"=→"Grabbing":bool, "Acq Control.Grab"=→"Acq Control.Grab":bool, "Acq Status.FrameHeight"=→"Acq Status.FrameHeight":u32, "Acq Status.FrameWidth"=→"Acq Status.FrameWidth":u32, "Timed Out?"=→"Timed Out?":bool, "AcqStatus.BufferToHostFull"=→"BufferToHost\\Full":bool, "AcqStatus.PushedToMem"=→"PushedToMem":u32, "AcqStatus.PushedToHost"=→"PushedToHost":u32, "AcqStatus.DataAvailable"=→"DataAvailable":u32, "AcqStatus.TenFrameTime"=w498:u32)  [unwired: 1 in, 1 out]
    "DMA Write Timeout?" <- w511
    "TenFrameTime" <- w498
    n225 = And(x=FALSE, y=w511) -> (x .and. y?=w509:bool)
    n226 = Multiply(x=1e-07, y=w498) -> (x*y=w496:dbl)
    n227 = case shown="True" w509 {
      tunnel: w522 -> [w532 _]
      tunnel: [w532 errorcluster {"status"=TRUE, "code"=-1, "source"="The write operation to the DMA FIFO on the FPGA timed out.  This can be caused by the DMA FIFO not being started or the DMA FIFO overflowing.  Make sure that Start is being called on the DMA FIFO.  Also make sure that the host application is reading from the DMA FIFO fast enough to prevent it from overflowing."} ("error out")] -> w521
      frame False {
      }
      frame True {
      }
    }
    n228 = Reciprocal(x=w496) -> (1/x=→"RealRate":dbl)
    n229 = flat-sequence {
      tunnel: w521 -> [w531]
      tunnel: [w529] -> w520
      frame #0 {
        n230 = Unbundle By Name(w531) -> ("status"=w530:bool)
        n231 = Or(x=w530, y="stopped") -> (x .or. y?=w529:bool)
        n232 = local write "stopped"(w529) -> ()
      }
    }
    "MonLoop" <- w514
  }
  n233 = while {
    tunnel: w49 -> [w536]
    stop <- w535 stop-if-true
    n234 = event shown="[1] \"Track\": Value Change" {
      selector: _ -> [_ _ _]
      dyn-events: _ -> [_ _ _]
      timeout: 50 -> [_ _ _]
      tunnel: w536 -> [w540 w557 _]
      event "Send": Value Change {
        n235 = event-data() -> ("NewVal"=w539:bool)  [unwired: 1 in, 4 out]
        n236 = Equal?(x=TRUE, y=w539) -> (x = y?=w537:bool)
        n237 = case shown="True" w537 {
          tunnel: w540 -> [_ w545]
          frame False {
          }
          frame True {
            n238 = Concatenate Strings("Command", "\r", "\n") -> (w542:string)
            n239 = call "WriteStringUART.vi"("String"=w542, "FPGA VI Reference In"=w545) -> ()  [unwired: 8 in, 2 out]
          }
        }
      }
      event "Track": Value Change {
        n240 = event-data() -> ("NewVal"=w546:bool)  [unwired: 1 in, 4 out]
        "Tracking" <- w546
        n241 = Equal?(x=w546, y=TRUE) -> (x = y?=w558:bool)
        n242 = case shown="True" w558 {
          tunnel: ["wse 0 1 0 0 1400 1024\r\nsot 80\r\n" w569] -> w556
          tunnel: [50.0 ("FrameRate") w568] -> w548
          tunnel: "FrameRate" -> [_ w568]
          tunnel: [25 5] -> w547
          frame False {
            (unwired) "wse 0 1 0 0 1024 800\r\nsot 80\r\n"
          }
          frame True {
            n243 = property on="Image" class="ImageControl"() -> ("ROI"=w576:T8)  [unwired: 2 in, 2 out]
            n244 = Unbundle By Name(w576) -> ("Global Rectangle"=w573:i32[])
            n245 = Index Array(array=w573, index #1=0 ("index"), index #2=1 ("index"), index #3=2 ("index"), index #4=3 ("index")) -> (element #1=w565:i32, element #2=w563:i32, element #3=w566:i32, element #4=w564:i32)
            n246 = Format Into String(format string="wse 0 1 %u %u %u %u\r\nsot 160\r\n", w565, w563, w566, w564) -> (resulting string=w569:string)  [unwired: 2 in, 1 out]
          }
        }
        n247 = Reciprocal(x=w548) -> (1/x=w551:dbl)
        n248 = local write "Viewing Rate"(w547) -> ()
        n249 = Multiply(x=w551, y=1000000.0) -> (x*y=w549:dbl)
        n250 = Format Into String(format string="set %u\rssf %u\r", w549, w548) -> (resulting string=w553:string)  [unwired: 2 in, 1 out]
        n251 = Concatenate Strings(w556, w553) -> (w555:string)
        n252 = call "WriteStringUART.vi"("String"=w555, "FPGA VI Reference In"=w557) -> ()  [unwired: 8 in, 2 out]
      }
      event Timeout {
        n253 = event-data() -> ()  [unwired: 1 in, 2 out]
      }
    }
    n254 = local read "stopped"() -> (w535:bool)
  }
  n255 = case shown="True" FALSE ("Start Serial Server?") {
    tunnel: w49 -> [_ w577]
    tunnel: [_ w578] -> w80
    frame False {
    }
    frame True {
      n256 = control-ref of="stopped"() -> (w579:refnum<vi>)
      n257 = call "SerialServer.vi"("Stop Refnum"=w579, "FPGA VI Reference In"=w577) -> ("FPGA VI Reference Out"=w578:refnum<k20>)  [unwired: 5 in]
    }
  }
  n258 = call <vilib>:"DAQmx Clear Task.vi"("task in"=w45) -> ("error out"=w23:errorcluster)  [unwired: 14 in]
  n259 = property on="Record" class="Bool (strict)"(error in=w23, "DisabledEnum"=w1) -> (error out=w24:errorcluster)  [unwired: 1 in, 1 out]
  n260 = property on="Calibration" class="Bool (strict)"(error in=w24, "DisabledEnum"=w1) -> (error out=w5:errorcluster)  [unwired: 1 in, 1 out]
  n261 = property on="Raw  Image" class="Bool (strict)"(error in=w5, "DisabledEnum"=w1) -> (error out=w2:errorcluster)  [unwired: 1 in, 1 out]
  n262 = property on="DA Output Task" class="DAQmxName (strict)"(error in=w2, "DisabledEnum"=w1) -> ()  [unwired: 1 in, 2 out]
  n263 = case shown="True" w12 {
    tunnel: w11 -> [_ w582]
    tunnel: w16 -> [_ w581]
    tunnel: w15 -> [_ w580]
    frame False {
    }
    frame True {
      n264 = call <instrlib>:"niHWS Close File.vi"("file handle"=w580) -> ()  [unwired: 10 in, 1 out]
      n265 = Close File(refnum=w581) -> ()  [unwired: 1 in, 2 out]
      n266 = call "IMAQ AVI Close"("Avi Refnum"=w582) -> ()  [unwired: 10 in, 1 out]
    }
  }
  n267 = stacked-sequence {
    tunnel: w18 -> [_ w584]
    frame #0 {
      n268 = Wait Until Next ms Multiple(millisecond multiple=u32 100) -> ()  [unwired: 1 out]
    }
    frame #1 {
      n269 = Release Queue(queue=w584) -> ()  [unwired: 2 in, 3 out]
    }
  }
  n270 = Merge Errors(w69, w68) -> (w70:errorcluster)
  n271 = flat-sequence {
    tunnel: w70 -> [w587]
    tunnel: [w587] -> w84
    tunnel: w82 -> [w586]
    tunnel: w80 -> [_]
    tunnel: w9 -> [w585]
    frame #0 {
      n272 = call "IMAQ Dispose"("Image"=w586) -> ()  [unwired: 5 in, 1 out]
      n273 = call "IMAQ Dispose"("Image"=w585) -> ()  [unwired: 5 in, 1 out]
    }
  }
  n274 = xnode "Close FPGA VI Reference"("FPGA VI Reference In"=w87, "error in"=w84) -> ("error out"=w81:errorcluster)
  n275 = call <vilib>:"Simple Error Handler.vi"("error in (no error)"=w81) -> ()  [unwired: 4 in, 5 out]
